vi "All Sorts.vi"() -> ()   [LabVIEW 2013]
panel:
  in  "Algorithm":string(combo)
  in  "Length":i32=50
  in  "Max":dbl=1024.0
  in  "Generate":bool
  out "Output":dbl[](array[numeric])
  in  "Input":dbl[](array[numeric])
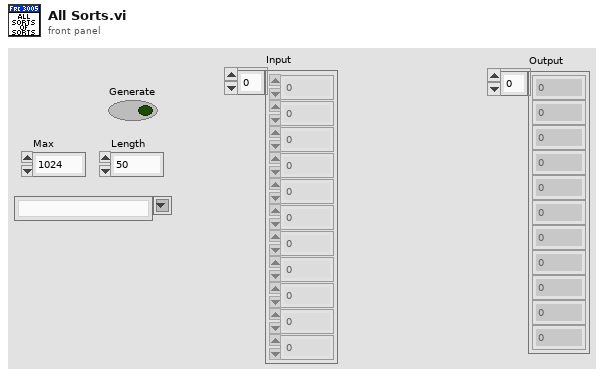
[diagram p1: front panel]
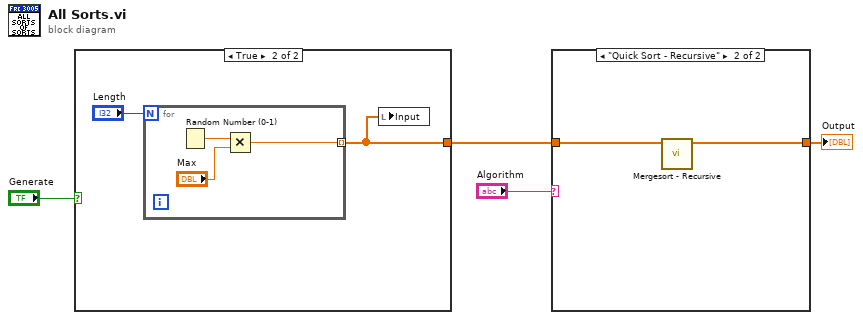
[diagram p0: block diagram]
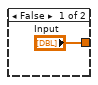
[diagram p3: hidden frame]
diagram:
  n1 = case shown="True" "Generate" {
    tunnel: ["Input" w6] -> w3
    frame False {
    }
    frame True {
      n2 = for {
        N: "Length" -> [_]
        tunnel: [w9] -> w6 mode=indexing
        n3 = Random Number (0-1)() -> (number: 0 to 1=w10:dbl)
        n4 = Multiply(x=w10, y="Max") -> (x*y=w9:dbl)
      }
      n5 = local write "Input"(w6) -> ()
    }
  }
  n6 = case shown="\"Quick Sort - Recursive\"" "Algorithm" {
    tunnel: w3 -> [w11 w13]
    tunnel: [w11 w12] -> w2
    frame Default {
    }
    frame "Quick Sort - Recursive" {
      n7 = call "Mergesort - Recursive.vi"("Input"=w13) -> ("Output"=w12:dbl[])  [unwired: 10 in]
    }
  }
  "Output" <- w2
